vi "FluxRead.vi"(3 "Error In":errorcluster, 4 "Função de Leitura":i32(ring)=2 items=["Zero in progress", "Perform flowmeter zeroing", "Mass flow rate", "Density", "Temperature", "Volume flow rate", "Pressure (internally derived)", "Mass total", "Volume total", "Mass inventory", "Volume inventory", "Start/stop all totalizers", "Reset all totalizers", "Reset all inventories", "Real-time interrupt failure", "Sensor failure", "Temperature sensor failure", "Flowmeter zeroing failure", "Other failure occurred", "Mass flow rate meter factor", "Volume flow rate meter factor", "Density meter factor", "Flowing density calibration constant", "Mass flow scale factor", "Density scale factor", "Temperature scale factor", "Volume flow scale factor", "Pressure scale factor", "Mass total scale factor", "Volume total scale factor", "Mass inventory scale factor", "Volume inventory scale factor", "Flowmeter zeroing standard deviantion (units in microsec)", "Standard or special mass flow unit", "Density unit", "Temperature unit", "Standard or special volume flow unit", "Pressure unit", "Standard or special mass total or inventory unit", "Standard or special volume total or inventory unit", "Base mass unit for special mass unit", "Base time uni for special mass unit", "Base volume unit for special volume unit", "Base time unit for special volume unit", "Maximum zeroing time", "Flow direction", "EEProm checksum failure", "EEProm checksum failure in core processor", "EEProm database corrupt", "RAM diagnostic failure", "RAM diagnostic failure in core processor", "Real-time Interrupt failure", "Watchdog timer error", "Mass flow cutoff", "Volume flow cutoff", "Integer de erro 001", "Slug flow high-density limit (g/cm3)", "Slug flow low-density limit (g/cm3)"], 5 "Master In":refnum<class "Modbus Master.lvclass">) -> (0 "Error Out":errorcluster, 1 "Data":dbl, 2 "Master Out":refnum<class "Modbus Master.lvclass">)   [LabVIEW 2019]
uses:
  <vilib>/Modbus/master/Modbus Master.lvclass
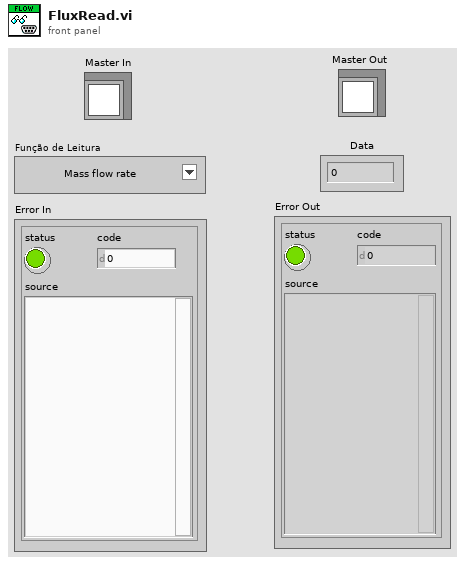
[diagram p1: front panel]
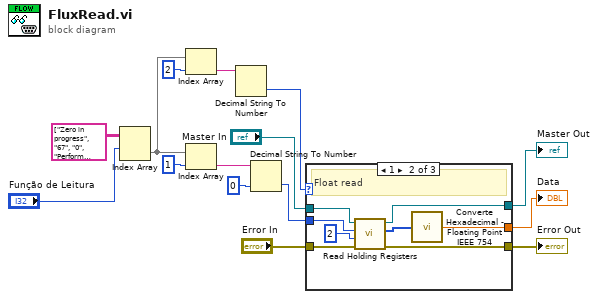
[diagram p0: block diagram]
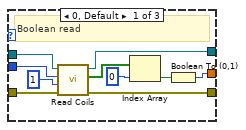
[diagram p2: hidden frame]
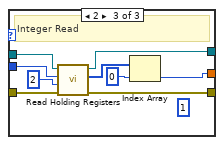
[diagram p3: hidden frame]
diagram:
  n1 = Index Array(array=string[][] [["Zero in progress", "67", "0"], ["Perform flowmeter zeroing", "4", "0"], ["Mass flow rate", "246", "1"], ["Density", "248", "1"], ["Temperature", "250", "1"], ["Volume flow rate", "252", "1"], ["Pressure (internally derived)", "256", "1"], ["Mass total", "258", "1"], ["Volume total", "260", "1"], ["Mass inventory", "262", "1"], ["Volume inventory", "264", "1"], ["Start/stop all totalizers", "1", "0"], ["Reset all totalizers", "2", "0"], ["Reset all inventories", "3", "0"], ["Real-time interrupt failure", "22", "0"], ["Sensor failure", "23", "0"], ["Temperature sensor failure", "24", "0"], ["Flowmeter zeroing failure", "25", "0"], ["Other failure occurred", "26", "0"], ["Mass flow rate meter factor", "278", "1"], ["Volume flow rate meter factor", "280", "1"], ["Density meter factor", "282", "1"], ["Flowing density calibration constant", "302", "1"], ["Mass flow scale factor", "28", "2"], ["Density scale factor", "29", "2"], ["Temperature scale factor", "30", "2"], ["Volume flow scale factor", "31", "2"], ["Pressure scale factor", "33", "2"], ["Mass total scale factor", "34", "2"], ["Volume total scale factor", "35", "2"], ["Mass inventory scale factor", "36", "2"], ["Volume inventory scale factor", "37", "2"], ["Flowmeter zeroing standard deviantion (units in microsec)", "230", "1"], ["Standard or special mass flow unit", "38", "2"], ["Density unit", "39", "2"], ["Temperature unit", "40", "2"], ["Standard or special volume flow unit", "41", "2"], ["Pressure unit", "43", "2"], ["Standard or special mass total or inventory unit", "44", "2"], ["Standard or special volume total or inventory unit", "45", "2"], ["Base mass unit for special mass unit", "131", "2"], ["Base time uni for special mass unit", "132", "2"], ["Base volume unit for special volume unit", "133", "2"], ["Base time unit for special volume unit", "134", "2"], ["Maximum zeroing time", "135", "2"], ["Flow direction", "16", "2"], ["EEProm checksum failure", "20", "0"], ["EEProm checksum failure in core processor", "418", "1"], ["EEProm database corrupt", "421", "1"], ["RAM diagnostic failure", "21", "0"], ["RAM diagnostic failure in core processor", "124", "1"], ["Real-time Interrupt failure", "22", "0"], ["Watchdog timer error", "32", "0"], ["Mass flow cutoff", "194", "1"], ["Volume flow cutoff", "196", "1"], ["Integer de erro 001", "0", "2"], ["Slug flow high-density limit (g/cm3)", "198", "1"], ["Slug flow low-density limit (g/cm3)", "200", "1"]] ("Tabela de funções de leitura"), index (row)="Função de Leitura") -> (element=w11:string[])  [unwired: 1 in]
  n2 = Index Array(array=w11, index=2) -> (element=w13:string)
  n3 = Index Array(array=w11, index=1) -> (element=w12:string)
  n4 = Decimal String To Number(string=w13) -> (number=w9:i32)  [unwired: 2 in, 1 out]
  n5 = Decimal String To Number(string=w12, default (0L)=u16 0 ("default (0 I32)")) -> (number=w8:u16)  [unwired: 1 in, 1 out]
  n6 = case shown="1" w9 {
    tunnel: "Master In" -> [w24 w33 w41]
    tunnel: "Error In" -> [w21 w29 w39]
    tunnel: [w20 w30 w38] -> w3
    tunnel: w8 -> [w17 w26 w35]
    tunnel: [w23 w32 w37] -> w2
    tunnel: [w19 w28 w36] -> w1
    frame 0, Default {
      # "Boolean read"
      n7 = call-dynamic "Read Coils.vi"("error in (no error)"=w21, "number of coils"=u16 1, "starting address"=w17, "Modbus master in"=w24) -> ("error out"=w20:errorcluster, "coil values"=w22:bool[], "Modbus master out"=w23:refnum<class "Modbus Master.lvclass">)  [unwired: 5 in]
      n8 = Index Array(array=w22, index=0) -> (element=w18:bool)
      n9 = Boolean To (0,1)(Boolean=w18) -> (0, 1=w19:i16)
    }
    frame 1 {
      # "Float read"
      n10 = call-dynamic "Read Holding Registers.vi"("error in (no error)"=w29, "number of holding registers"=u16 2 ("Quantity"), "starting address"=w26, "Modbus master in"=w33) -> ("error out"=w30:errorcluster, "register values"=w31:u16[], "Modbus master out"=w32:refnum<class "Modbus Master.lvclass">)  [unwired: 5 in]
      n11 = call "Converte Hexadecimal - Floating Point IEEE 754.vi"("Par de registradores"=w31) -> ("Floating point"=w28:sgl)
    }
    frame 2 {
      (unwired) u16 1 ("read operation starting address")
      # "Integer Read"
      n12 = call-dynamic "Read Holding Registers.vi"("error in (no error)"=w39, "number of holding registers"=u16 2, "starting address"=w35, "Modbus master in"=w41) -> ("error out"=w38:errorcluster, "register values"=w40:u16[], "Modbus master out"=w37:refnum<class "Modbus Master.lvclass">)  [unwired: 5 in]
      n13 = Index Array(array=w40, index=0) -> (element=w36:u16)
    }
  }
  "Master Out" <- w2
  "Error Out" <- w3
  "Data" <- w1
